vi "Execute.vi"(8 "error in (no error)":errorcluster, 11 "reference in":refnum<class "CeilingFanHighCommand.lvclass">) -> (0 "error out":errorcluster, 3 "reference in":refnum<class "CeilingFanHighCommand.lvclass">)   [LabVIEW 2020, in "CeilingFanHighCommand.lvclass"]
uses:
  CeilingFanHighCommand.lvclass
  CeilingFan_class/CeilingFan.lvclass
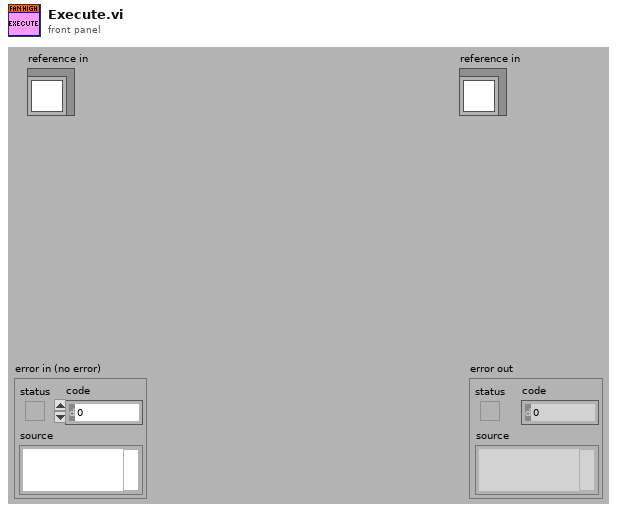
[diagram p1: front panel]
types:
  T1 = typedef "CeilingFanHighCommand.lvclass/ObjectAttributes.ctl" = cluster{"CeilingFan":refnum<class "CeilingFan.lvclass">, "PrevSpeed":i32}
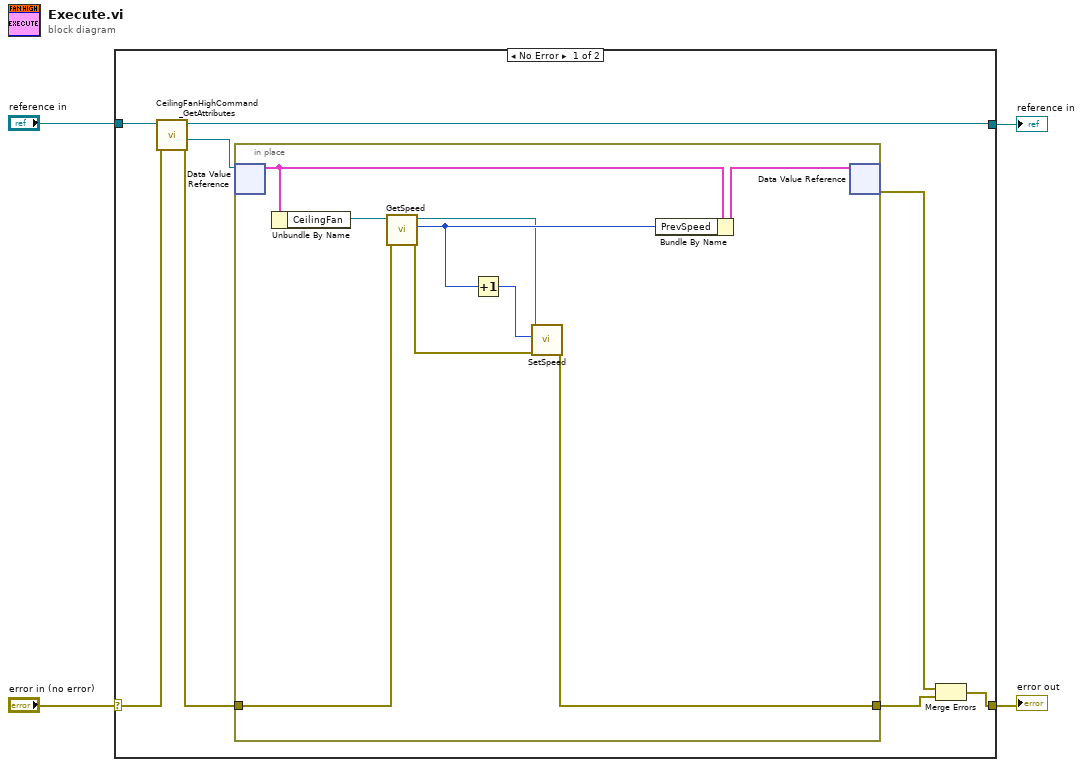
[diagram p0: block diagram]
diagram:
  n1 = case shown="No Error" "error in (no error)" {
    selector: "error in (no error)" -> [w11 w23]
    tunnel: [w9 w23] -> w3
    tunnel: [w8 w22] -> w1
    tunnel: "reference in" -> [w12 w22]
    frame No Error {
      n2 = call "CeilingFanHighCommand_GetAttributes.vi"("error in (no error)"=w11, "reference in"=w12) -> ("error out"=w6:errorcluster, "DataRef"=w7:refnum<data-value>, "reference out"=w8:refnum<class "CeilingFanHighCommand.lvclass">)  [unwired: 6 in, 1 out]
      n3 = in-place {
        in-place-border: w6 -> [w14]
        in-place-border: [w13] -> w5
        n4 = in-place-dvr #1(w7) -> (w20:T1)  [unwired: 1 out]
        n5 = Unbundle By Name(w20) -> ("CeilingFan"=w19:refnum<class "CeilingFan.lvclass">)
        n6 = call-dynamic "GetSpeed.vi"("error in (no error)"=w14, "reference in"=w19) -> ("error out"=w18:errorcluster, "Speed"=w17:i32, "reference out"=w15:refnum<class "CeilingFan.lvclass">)  [unwired: 7 in]
        n7 = Increment(x=w17) -> (x+1=w16:i32)
        n8 = call-dynamic "SetSpeed.vi"("error in (no error)"=w18, "Speed"=w16, "reference in"=w15) -> ("error out"=w13:errorcluster)  [unwired: 7 in, 1 out]
        n9 = Bundle By Name(cluster=w20, "PrevSpeed"=w17) -> (w21:T1)
        n10 = in-place-dvr #1(w21) -> (w10:errorcluster)  [unwired: 1 out]
      }
      n11 = Merge Errors(w10, w5) -> (w9:errorcluster)
    }
    frame Error {
    }
  }
  "error out" <- w3
  "reference in" <- w1
